vi "aaa1.vi"() -> ()   [LabVIEW 2010]
uses:
  <vilib>/Utility/miscctls.llb/LVBoundsTypeDef.ctl
  <vilib>/Utility/miscctls.llb/LVKeyTypeDef.ctl
  <vilib>/Utility/miscctls.llb/LVSelectionTypeDef.ctl
  <vilib>/Utility/miscctls.llb/LVStringsAndValuesArrayTypeDef.ctl
panel:
  in  "Ring":u16(ring) items=["gas flow: off", "rus loop: on", "rus loop: off", "itc box: off", "itc box: heater manual and zero", "itc box: gas zero", "itc box: read state", "itc box: heater auto", "itc box: set temperature to \\d+", "itc box: set temperature to", "gas flow: on", "gas flow: force up", "gas flow: force down", "gas flow: stop up/down", "gas flow: set to \\d+", "gas rus itc: stop", "tabs: disable", "tabs: enable", "all: init"]
  out "Strings []":string[](array[string])
  in  "action":T1(ring)=enum."check"
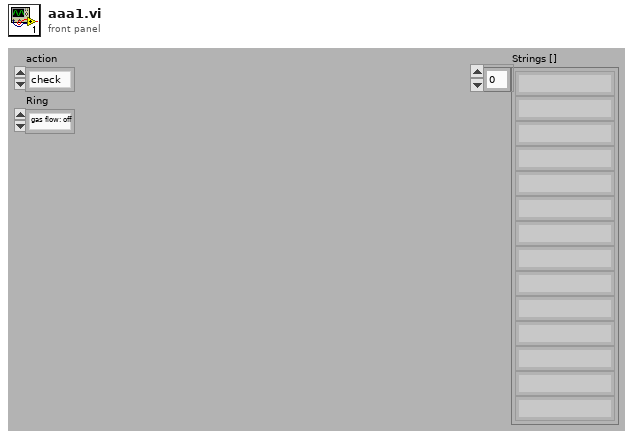
[diagram p1: front panel]
types:
  T1 = enum16{"init", "check", "reset", "log", "change path", "message"}
  T2 = typedef "LVStringsAndValuesArrayTypeDef.ctl" = cluster{"String":string, "Value":ext}[]
  T3 = typedef "LVSelectionTypeDef.ctl" = cluster{"Selection Start":u32, "Selection End":u32}
  T4 = typedef "LVKeyTypeDef.ctl" = cluster{"Focus":bool, "Control":bool, "Shift":bool, "Key":string}
  T5 = typedef "LVBoundsTypeDef.ctl" = cluster{"Width":u32, "Height":u32}
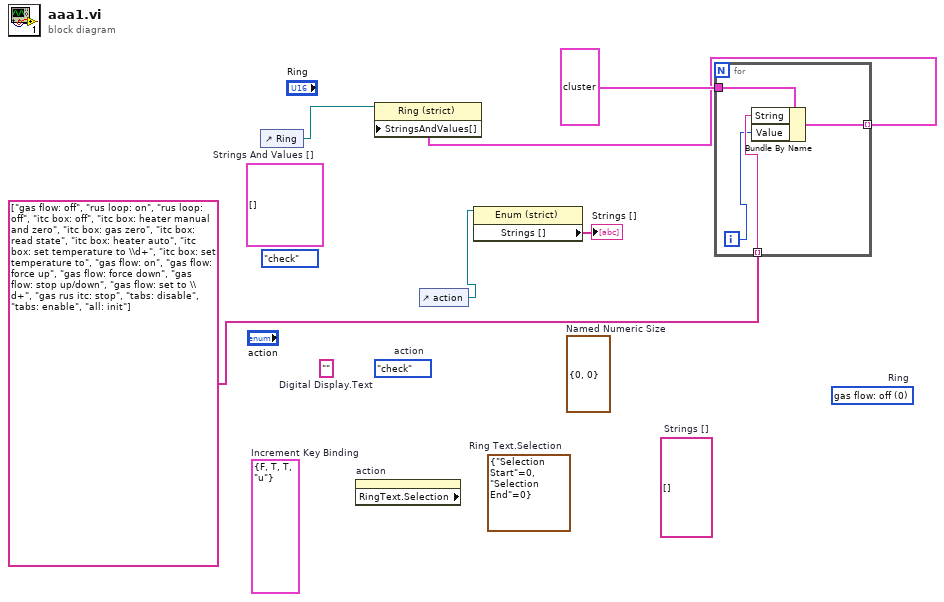
[diagram p0: block diagram]
diagram:
  (unwired) u16 0 items=["gas flow: off", "rus loop: on", "rus loop: off", "itc box: off", "itc box: heater manual and zero", "itc box: gas zero", "itc box: read state", "itc box: heater auto", "itc box: set temperature to \\d+", "itc box: set temperature to", "gas flow: on", "gas flow: force up", "gas flow: force down", "gas flow: stop up/down", "gas flow: set to \\d+", "gas rus itc: stop", "tabs: disable", "tabs: enable", "all: init"]  # Ring
  (unwired) T2 []  # Strings And Values []
  (unwired) string[] []  # Strings []
  (unwired) T3 {"Selection Start"=0, "Selection End"=0}  # Ring Text.Selection
  (unwired) T4 {"Focus"=FALSE, "Control"=TRUE, "Shift"=TRUE, "Key"="u"}  # Increment Key Binding
  (unwired) T1."check"  # action
  (unwired) ""  # Digital Display.Text
  (unwired) T5 {"Width"=0, "Height"=0}  # Named Numeric Size
  (unwired) T1."check" ("action")
  n1 = control-ref of="Ring"() -> (w6:refnum<vi>)
  n2 = property on="action" class="Enum (strict)" props=["RingText", "Selection"]() -> ()  [unwired: 2 in, 3 out]
  n3 = control-ref of="action"() -> (w1:refnum<vi>)
  n4 = property class="Enum (strict)"(reference=w1) -> ("Strings []"=→"Strings []":string[])  [unwired: 1 in, 2 out]
  n5 = for {
    tunnel: string[] ["gas flow: off", "rus loop: on", "rus loop: off", "itc box: off", "itc box: heater manual and zero", "itc box: gas zero", "itc box: read state", "itc box: heater auto", "itc box: set temperature to \\d+", "itc box: set temperature to", "gas flow: on", "gas flow: force up", "gas flow: force down", "gas flow: stop up/down", "gas flow: set to \\d+", "gas rus itc: stop", "tabs: disable", "tabs: enable", "all: init"] -> [w9] mode=indexing
    tunnel: cluster{"String":string, "Value":ext} {"String"="", "Value"=0.0} -> [w10]
    tunnel: [w8] -> w3 mode=indexing
    i -> [w7]
    n6 = Bundle By Name(cluster=w10, "String"=w9, "Value"=w7) -> (w8:cluster{"String":string, "Value":ext})
  }
  n7 = property class="Ring (strict)"(reference=w6, "StringsAndValues[]"=w3) -> ()  [unwired: 1 in, 2 out]
